vi "Read Init.vi"(8 "error in (no error)":errorcluster, 11 "Vapour Generator in":refnum<class "Vapour Generator.lvclass">) -> (0 "error out":errorcluster, 2 "Init":bool, 3 "Vapour Generator out":refnum<class "Vapour Generator.lvclass">)   [LabVIEW 2011, in "Vapour Generator.lvclass"]
uses:
  Vapour Generator.lvclass
  Vapour Generator.lvclass/Vapour Generator.ctl
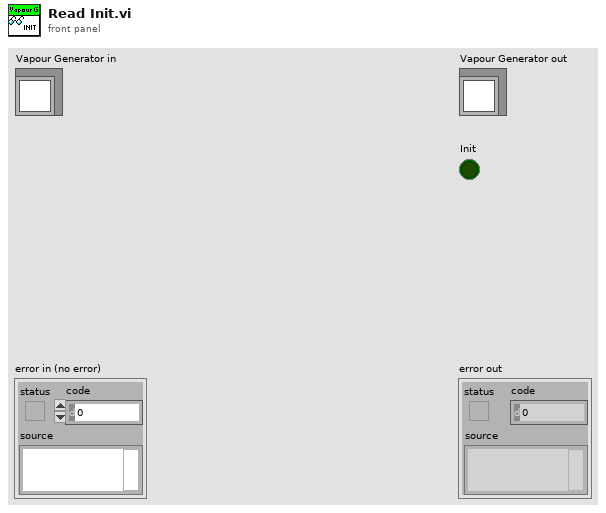
[diagram p1: front panel]
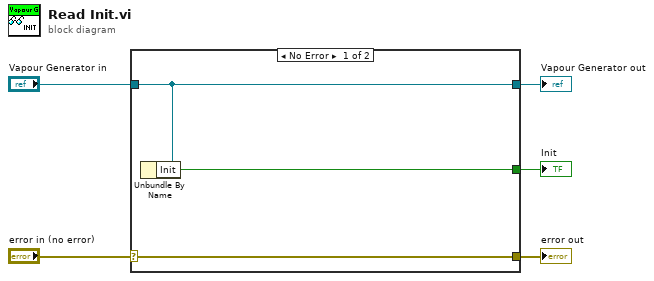
[diagram p0: block diagram]
diagram:
  n1 = case shown="No Error" "error in (no error)" {
    selector: "error in (no error)" -> [w8 w9]
    tunnel: [w8 w9] -> w4
    tunnel: [w7 w10] -> w2
    tunnel: "Vapour Generator in" -> [w7 w10]
    tunnel: [w6 _] -> w1
    frame No Error {
      n2 = Unbundle By Name(w7) -> ("Init"=w6:bool)
    }
    frame Error {
    }
  }
  "error out" <- w4
  "Vapour Generator out" <- w2
  "Init" <- w1
